vi "Get Measurement Configuration Controls.vi"(7 "error in":errorcluster, 10 "measurement configuration control path":path) -> (0 "error out":errorcluster, 3 "controls":refnum<vi>[](array[refnum]))   [LabVIEW 2021, in "NI Measurement Plug-In SDK.lvlib"]
uses:
  NI Measurement Plug-In SDK.lvlib
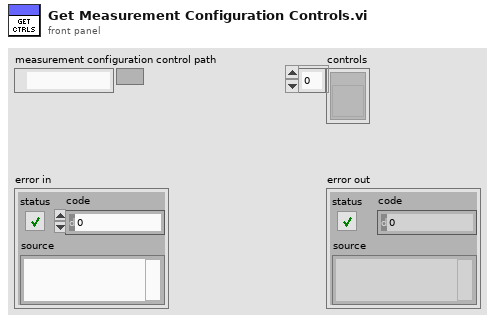
[diagram p1: front panel]
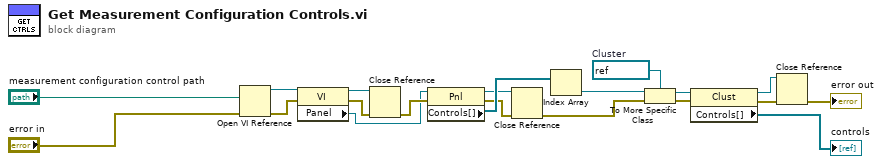
[diagram p0: block diagram]
diagram:
  w17 = refnum<vi> refnum  # Cluster
  n1 = Open VI Reference(vi path="measurement configuration control path", error in (no error)="error in") -> (vi reference=w11:refnum<vi>, error out=w19:errorcluster)  [unwired: 4 in]
  n2 = property class="VI"(reference=w11, error in=w19) -> (reference out=w15:refnum<vi>, error out=w13:errorcluster, "Panel"=w12:refnum<vi>)
  n3 = Close Reference(reference=w15, error in (no error)=w13) -> (error out=w14:errorcluster)
  n4 = property class="Pnl"(reference=w12, error in=w14) -> (reference out=w3:refnum<vi>, error out=w5:errorcluster, "Controls[]"=w20:refnum<vi>[])
  n5 = Close Reference(reference=w3, error in (no error)=w5) -> (error out=w4:errorcluster)
  n6 = Index Array(array=w20) -> (element=w18:refnum<vi>)  [unwired: 1 in]
  n7 = To More Specific Class(target class=w17, reference=w18, error in=w4) -> (specific class reference=w16:refnum<vi>, error out=w10:errorcluster)
  n8 = property class="Clust"(reference=w16, error in=w10) -> (reference out=w6:refnum<vi>, error out=w8:errorcluster, "Controls[]"=→"controls":refnum<vi>[])
  n9 = Close Reference(reference=w6, error in (no error)=w8) -> (error out=→"error out":errorcluster)
